vi "Monitor.vi"() -> ()   [LabVIEW 2017]
uses:
  <vilib>/Motion/Express/_s/nimc.fb.read.readExecutionData.axis.vi
  <vilib>/Motion/BlockNode/FB.NIMotion.xnode
panel:
  in  "Stop Button":bool
  in  "Tab Control":enum32{"Posición", "Velocidad"}(tab)
  out "Posición 2":dbl(graph)
  out "Posición 1":dbl(graph)
  out "Velocidad 2":dbl(graph)
  out "Velocidad 1":dbl(graph)
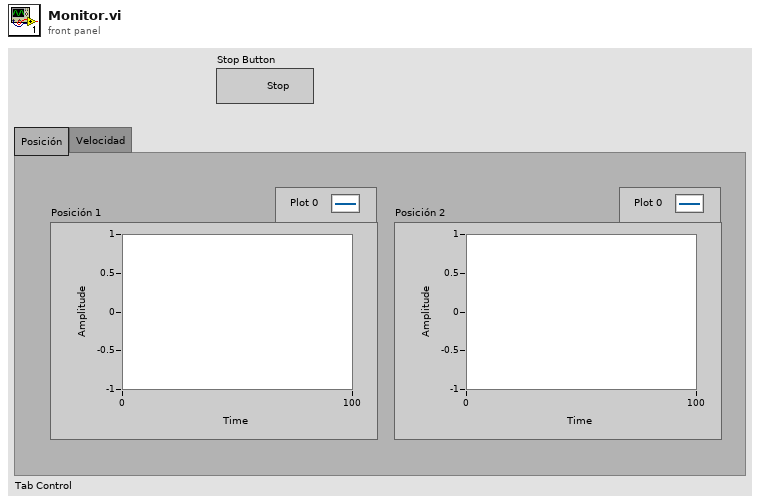
[diagram p1: front panel]
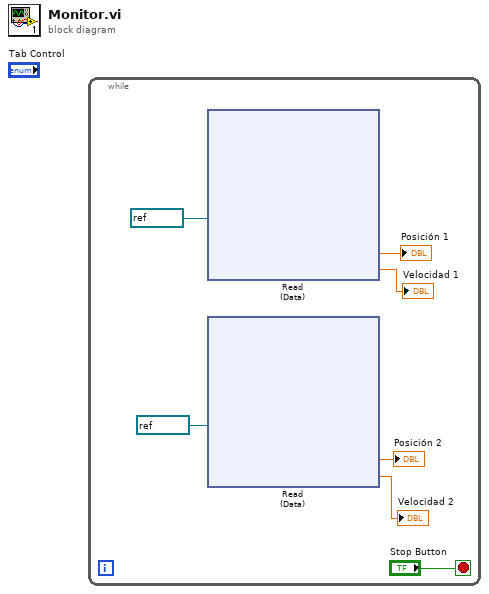
[diagram p0: block diagram]
diagram:
  n1 = while {
    stop <- "Stop Button" stop-if-true
    n2 = xnode "Read\n(Data)"("resource"=refnum<k21> "Eje X") -> ("position"=→"Posición 1":dbl, "velocity"=→"Velocidad 1":dbl)  [unwired: 1 in, 3 out]
    n3 = xnode "Read\n(Data)"("resource"=refnum<k21> "Eje Y") -> ("position"=→"Posición 2":dbl, "velocity"=→"Velocidad 2":dbl)  [unwired: 1 in, 3 out]
  }
